vi "Query Audio Devices.vi"(8 "error in (no error)":errorcluster, 11 "Backend (Default)":T3=enum."Default") -> (0 "error out":errorcluster, 1 "Loopback Devices":T1[](array[typedef]), 2 "Capture Devices":T1[](array[typedef]), 3 "Playback Devices":T1[](array[typedef]), 4 "Device Errors":errorcluster[](array[cluster]))   [LabVIEW 2020, in "G-Audio.lvlib"]
doc: "Query the available audio devices for playback, capture, and loopback. If Backend is specified, the audio devices for that backend are enumerated. Otherwise the devices for the default audio backend are enumerated.\n\n<b>Loopback Devices</b> is valid only if the backend is WASAPI, or the default backend is WASAPI. Other backends do not support loopback devices.\n\nOnly devices which didn't return an error are included in the outputs. Check Device Errors for any devices which may have errored.\n\n<b>WARNING: Do not call this function from a VI running with a Preferred Execution System of 'user interface'.</b>"
uses:
  G-Audio.lvlib
  Controls/Backends.ctl
  Controls/Audio Device Info.ctl
  Controls/Audio Device Type.ctl
  <vilib>/Utility/error.llb/Error Cluster From Error Code.vi
  lib/g_audio_32.dll
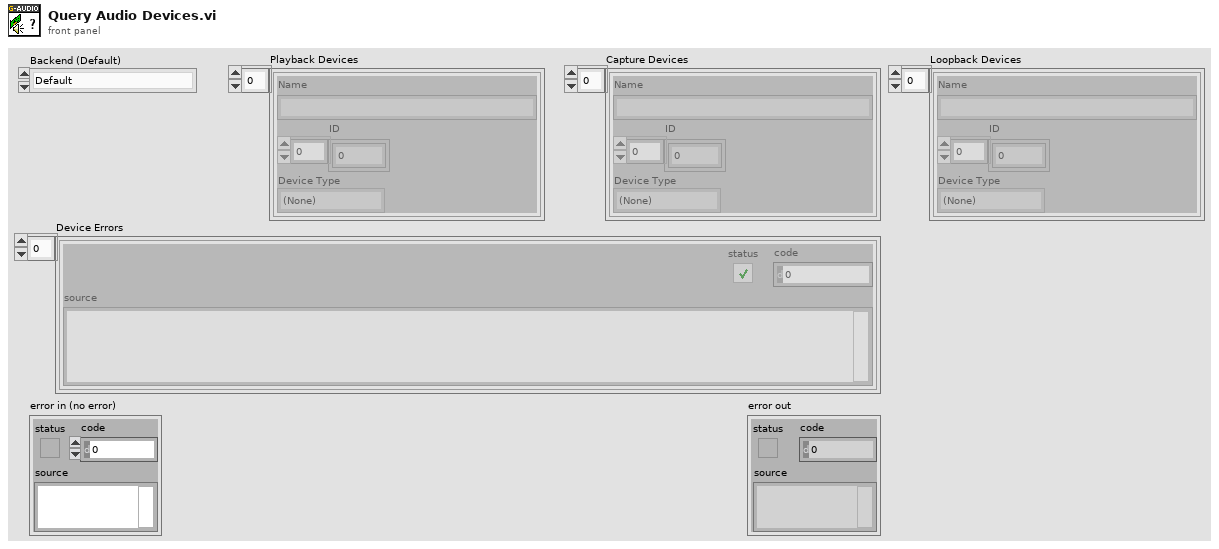
[diagram p1: front panel]
types:
  T1 = typedef "G-Audio.lvlib/Audio Device Info.ctl" = cluster{"Name":string, "ID":u8[], "Device Type":T2}
  T2 = typedef "G-Audio.lvlib/Audio Device Type.ctl" = enum16{"(None)", "Playback", "Capture", "Duplex", "Loopback"}
  T3 = typedef "G-Audio.lvlib/Backends.ctl" = enum16{"WASAPI", "DirectSound", "WinMM", "Core Audio", "sndio", "audio(4)", "OSS", "PulseAudio", "ALSA", "JACK", "AAudio", "OpenSL|ES", "Web Audio", "Custom", "Null", "Default"}
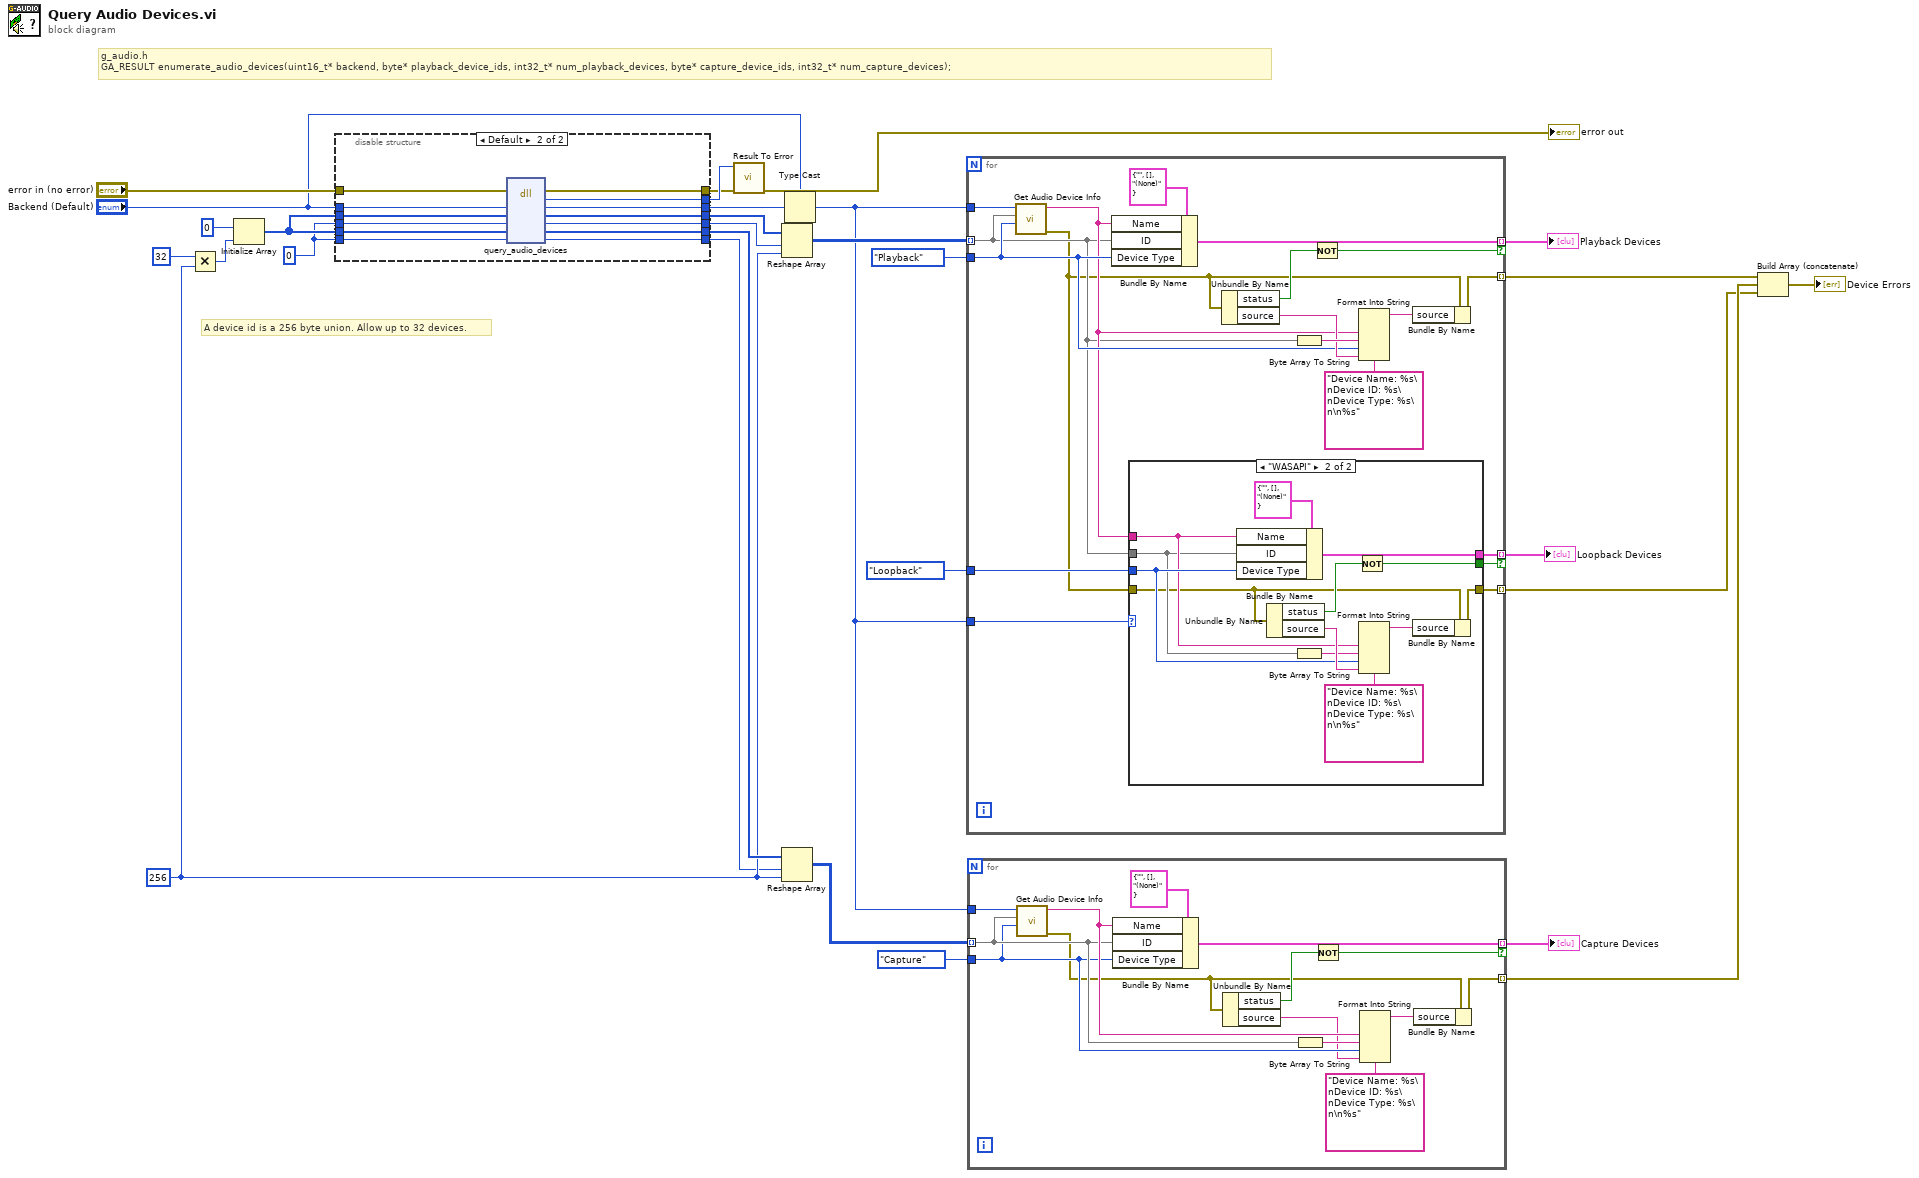
[diagram p0: block diagram]
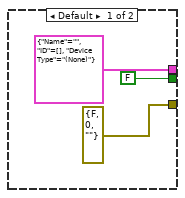
[diagram p2: hidden frame]
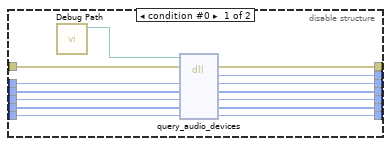
[diagram p3: hidden frame]
diagram:
  w22 = 0 ("num_playback_devices")
  w18 = 256
  # "A device id is a 256 byte union. Allow up to 32 devices."
  # "g_audio.h\nGA_RESULT enumerate_audio_devices(uint16_t* backend, byte* playback_device_ids, int32_t* num_playback_devices, byte* capture_device_ids, int32_t* num_capture_devices);"
  n1 = Multiply(x=32, y=w18) -> (x*y=w25:i32)
  n2 = Initialize Array(u8 0, w25) -> (w23:u8[])
  n3 = disable-structure shown="Default" {
    disable-tunnel: "error in (no error)" -> [w43 w56]
    disable-tunnel: "Backend (Default)" -> [w40 w53]
    disable-tunnel: [w42 w55] -> w28
    disable-tunnel: w23 -> [w37 w50]
    disable-tunnel: [w38 w51] -> w20
    disable-tunnel: [w41 w54] -> w29
    disable-tunnel: [w39 w52] -> w3
    disable-tunnel: w23 -> [w36 w49]
    disable-tunnel: w22 -> [w35 w48]
    disable-tunnel: w22 -> [w34 w47]
    disable-tunnel: [w33 w46] -> w19
    disable-tunnel: [w32 w45] -> w21
    disable-tunnel: [w31 w44] -> w17
    frame condition #0 {
      n4 = call "Debug Path.vi"() -> ("Debug Path"=w30:path)  [unwired: 11 in]
      n5 = dll-call lib="?" fn="query_audio_devices"(path in=w30, error in=w43, "backend"=w40, "playback_device_ids"=w37, "num_playback_devices"=w35, "capture_device_ids"=w36, "num_capture_devices"=w34) -> (error out=w42:errorcluster, "result"=w41:i32, "backend"=w39:u16, "playback_device_ids"=w38:u8[], "num_playback_devices"=w33:i32, "capture_device_ids"=w32:u8[], "num_capture_devices"=w31:i32)  [unwired: 1 in, 1 out]
    }
    frame condition #1 (active) {
      n6 = dll-call lib="C:/github/dataflowg/g-audio/src/LabVIEW/G-Audio/lib/g_audio_*.*" fn="query_audio_devices"(error in=w56, "backend"=w53, "playback_device_ids"=w50, "num_playback_devices"=w48, "capture_device_ids"=w49, "num_capture_devices"=w47) -> (error out=w55:errorcluster, "result"=w54:i32, "backend"=w52:u16, "playback_device_ids"=w51:u8[], "num_playback_devices"=w46:i32, "capture_device_ids"=w45:u8[], "num_capture_devices"=w44:i32)  [unwired: 2 in, 1 out]
    }
  }
  n7 = call "Result To Error.vi"("error in (no error)"=w28, "Result Code"=w29) -> ("error out"=→"error out":errorcluster)  [unwired: 9 in]
  n8 = Reshape Array(w20, w19, w18) -> (w16:u8[][])
  n9 = Reshape Array(w21, w17, w18) -> (w11:u8[][])
  n10 = Type Cast(type="Backend (Default)", x=w3) -> (*(type *) &x=w2:T3)
  n11 = for {
    tunnel: w2 -> [w75]
    tunnel: w16 -> [w58] mode=indexing
    tunnel: [w73] -> w14 mode=indexing if=w71
    tunnel: Audio_Device_Type."Playback" ("Device Type (Playback)") -> [w61]
    tunnel: [w66] -> w10 mode=indexing
    tunnel: [w65] -> w4 mode=indexing
    tunnel: Audio_Device_Type."Loopback" ("Device Type (Playback)") -> [w64]
    tunnel: [w63] -> w5 mode=indexing if=w60
    tunnel: w2 -> [w62]
    n12 = call "Get Audio Device Info.vi"("Device Type (Playback)"=w61, "Playback Device ID"=w58, "Backend (Default)"=w75) -> ("error out"=w57:errorcluster, "Device Info"=w59:string)  [unwired: 7 in]
    n13 = Bundle By Name(cluster=T1 {"Name"="", "ID"=[], "Device Type"=enum."(None)"} ("Audio Device Info"), "Name"=w59, "ID"=w58, "Device Type"=w61) -> (w73:T1)
    n14 = case shown="\"WASAPI\"" w62 {
      tunnel: [errorcluster {"status"=FALSE, "code"=0, "source"=""} ("error out") w91] -> w65
      tunnel: w64 -> [_ w82]
      tunnel: [T1 {"Name"="", "ID"=[], "Device Type"=enum."(None)"} ("Audio Device Info") w84] -> w63
      tunnel: [FALSE w83] -> w60
      tunnel: w59 -> [_ w81]
      tunnel: w58 -> [_ w80]
      tunnel: w57 -> [_ w79]
      frame Default {
      }
      frame "WASAPI" {
        n15 = Bundle By Name(cluster=T1 {"Name"="", "ID"=[], "Device Type"=enum."(None)"} ("Audio Device Info"), "Name"=w81, "ID"=w80, "Device Type"=w82) -> (w84:T1)
        n16 = Unbundle By Name(w79) -> ("status"=w86:bool, "source"=w90:string)
        n17 = Byte Array To String(unsigned byte array=w80) -> (string=w88:string)
        n18 = Not(x=w86) -> (.not. x?=w83:bool)
        n19 = Format Into String(format string="Device Name: %s\nDevice ID: %s\nDevice Type: %s\n\n%s", w81, w88, w82, w90) -> (resulting string=w89:string)  [unwired: 2 in, 1 out]
        n20 = Bundle By Name(cluster=w79, "source"=w89) -> (w91:errorcluster)
      }
    }
    n21 = Unbundle By Name(w57) -> ("status"=w72:bool, "source"=w67:string)
    n22 = Byte Array To String(unsigned byte array=w58) -> (string=w69:string)
    n23 = Not(x=w72) -> (.not. x?=w71:bool)
    n24 = Format Into String(format string="Device Name: %s\nDevice ID: %s\nDevice Type: %s\n\n%s", w59, w69, w61, w67) -> (resulting string=w68:string)  [unwired: 2 in, 1 out]
    n25 = Bundle By Name(cluster=w57, "source"=w68) -> (w66:errorcluster)
  }
  "Playback Devices" <- w14
  "Loopback Devices" <- w5
  n26 = for {
    tunnel: w2 -> [w105]
    tunnel: w11 -> [w98] mode=indexing
    tunnel: [w103] -> w9 mode=indexing if=w101
    tunnel: Audio_Device_Type."Capture" ("Device Type (Playback)") -> [w96]
    tunnel: [w92] -> w8 mode=indexing
    n27 = call "Get Audio Device Info.vi"("Device Type (Playback)"=w96, "Playback Device ID"=w98, "Backend (Default)"=w105) -> ("error out"=w93:errorcluster, "Device Info"=w99:string)  [unwired: 7 in]
    n28 = Bundle By Name(cluster=T1 {"Name"="", "ID"=[], "Device Type"=enum."(None)"} ("Audio Device Info"), "Name"=w99, "ID"=w98, "Device Type"=w96) -> (w103:T1)
    n29 = Unbundle By Name(w93) -> ("status"=w102:bool, "source"=w94:string)
    n30 = Byte Array To String(unsigned byte array=w98) -> (string=w97:string)
    n31 = Not(x=w102) -> (.not. x?=w101:bool)
    n32 = Format Into String(format string="Device Name: %s\nDevice ID: %s\nDevice Type: %s\n\n%s", w99, w97, w96, w94) -> (resulting string=w95:string)  [unwired: 2 in, 1 out]
    n33 = Bundle By Name(cluster=w93, "source"=w95) -> (w92:errorcluster)
  }
  "Capture Devices" <- w9
  n34 = Build Array (concatenate)(w10, w8, w4) -> (→"Device Errors":errorcluster[])
